vi "Digital Twin UI.vi"(8 "error in (no error)":errorcluster) -> (0 "error out":errorcluster)   [LabVIEW 2018]
uses:
  <vilib>/robotics/Controls/Simulator Display/Simulator Display.xctl
  Source Code_Headless/TestExec.llb/State Selector.ctl
  <vilib>/robotics/Simulator/Engine/ctl/Step Mode.ctl
  Source Code_Headless/TestExec.llb/TestStand UI Data.ctl
  <vilib>/NI Veristand/Execution/Workspace/NI VeriStand - Get Multiple Channel Values.vi
  <instrlib>/DC Motor Controller/HAIOL/DC Motor Controller.lvclass
  <vilib>/robotics/Simulator/NI_Robotics_Simulator.lvlib
  <instrlib>/DC Motor Controller/HAIOL/Simulator/DC Motor Controller Simulator.lvclass
  Source Code_Headless/TestExec.llb/TestStand Simple UI Dependencies.lvlib
  <vilib>/NI Veristand/Execution/Workspace/NI_VS Workspace ExecutionAPI.lvlib
  <vilib>/vision/driver/NI_Vision_Acquisition_Software.lvlib
  <resource>/objmgr/imaqdx.rc
panel:
  out "Enum":T1
  in  "TestStand UI Button Control":refnum<k7>(container)
  out "Numeric 2":i32
  out "DemoStop":bool
  out "DemoStart":bool
  out "Numeric":i32
  out "读数停止":bool
  out "Real Gear Position":T2(plugin-control)
  out "Time Stamp Control":timestamp format="%<%Y/%m/%d %X>T"
  out "WFC":dbl[][](graph)
  out "WFC - error":dbl[][](graph)
  out "Real Gear Enabled":bool
  out "Command":u16(ring) items=["抬起，Up，↑↑↑", "放下，Down，↓↓↓", "关闭，close，→→→"]
  out "WFC - torque":dbl(graph)
  out "Position Error:":dbl format="%#g deg"
  out "Sim Gear N Position:":dbl format="%#g deg"
  out "Real Gear N Position:":dbl format="%#g deg"
  out "LGCU Torque DutyCycle:":dbl format="%#g"
  out "Bypass Torque Calibration":bool
  out "Bypass Position Calibration":bool
  out "Sim Gear Position [deg]":dbl(slide) scale=0.0..180.0
  in  "Application Manager":refnum<k7>(container)
  in  "SequenceFileView Manager":refnum<k7>(container)
  in  "ExecutionView Manager":refnum<k7>(container)
  in  "Simulator Display":refnum<vi>(xcontrol)
  in  "manifest filename":string="Robotics Environment Simulator.xml"
  # "Digital Twin Demo -- Landing Gear Test"
  # "Gear Model"
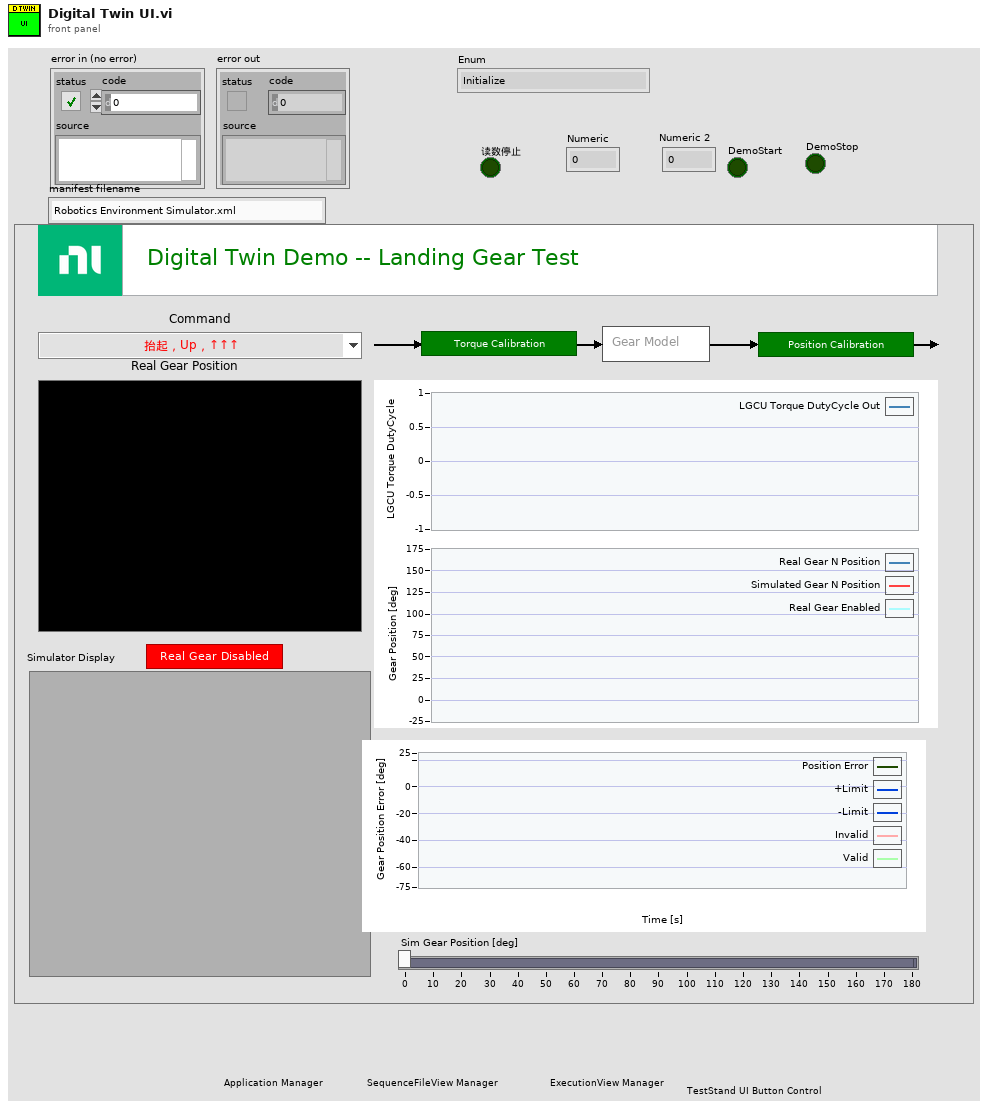
[diagram p1: front panel]
types:
  T1 = typedef "TestStand Simple UI Dependencies.lvlib/State Selector.ctl" = enum16{"Initialize", "Configure Connections", "Register Event Callbacks", "Start Application", "Execute", "Wait", "Stop", "Shutdown", "Handle Errors"}
  T2 = typedef "IMAQ Image.ctl" = refnum<image>
  T3 = typedef "TestStand Simple UI Dependencies.lvlib/TestStand UI Data.ctl" = cluster{"Other References":cluster{"Event Callback":refnum<k27>, "Quit Application Event":refnum<user-event>, "Event Reg Refnum":refnum<event-registration>, "Top level VI":refnum<vi>, "TestStand Engine":refnum<k7>}, "Manager Controls":cluster{"Application Manager":refnum<k7>, "SequenceFileView Manager":refnum<k7>, "ExecutionView Manager":refnum<k7>}, "Visible Controls":cluster{"Exit Button":refnum<k7>}}
  T4 = cluster{"Robot ID":string, "Device Label":string}
  T5 = typedef "NI_Robotics_Simulator.lvlib/Step Mode.ctl" = u16
  T6 = enum32{"invalid app kind", "Development System", "Run Time System", "Student Edition", "Embedded LabVIEW", "Evaluation", "Custom"}
  T7 = typedef "NI_VS Workspace ExecutionAPI.lvlib/WorkspaceAPI.ctl" = refnum<k24>
  T8 = typedef "IMAQdx.ctl" = refnum<k21>
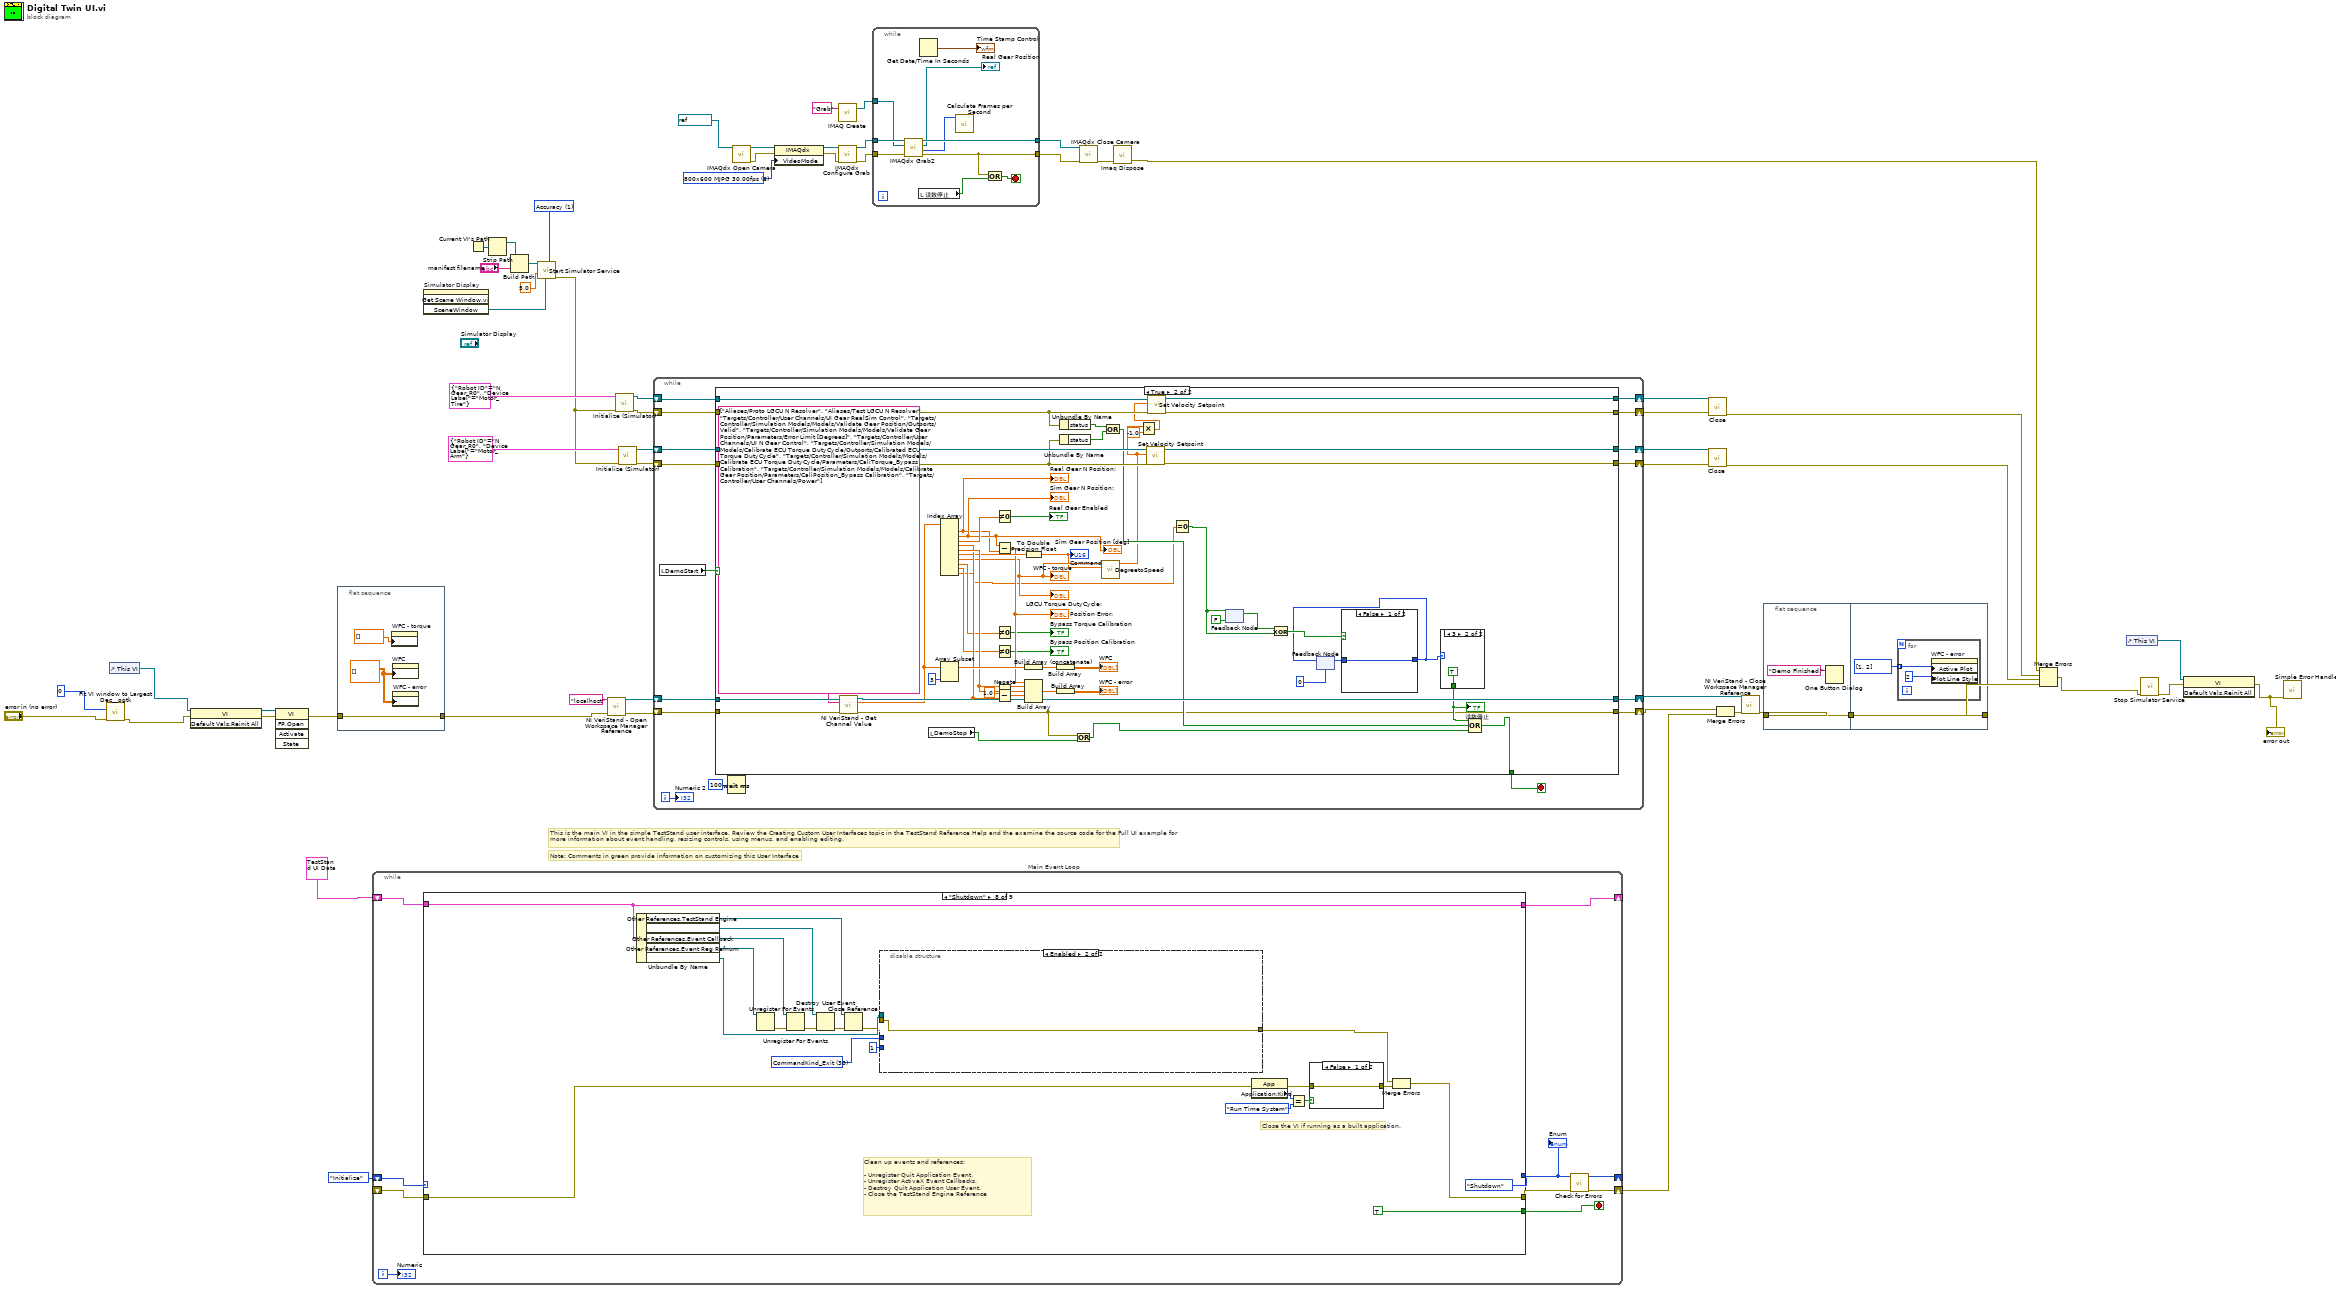
[diagram p0: block diagram]
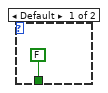
[diagram p3: hidden frame]
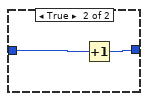
[diagram p4: hidden frame]
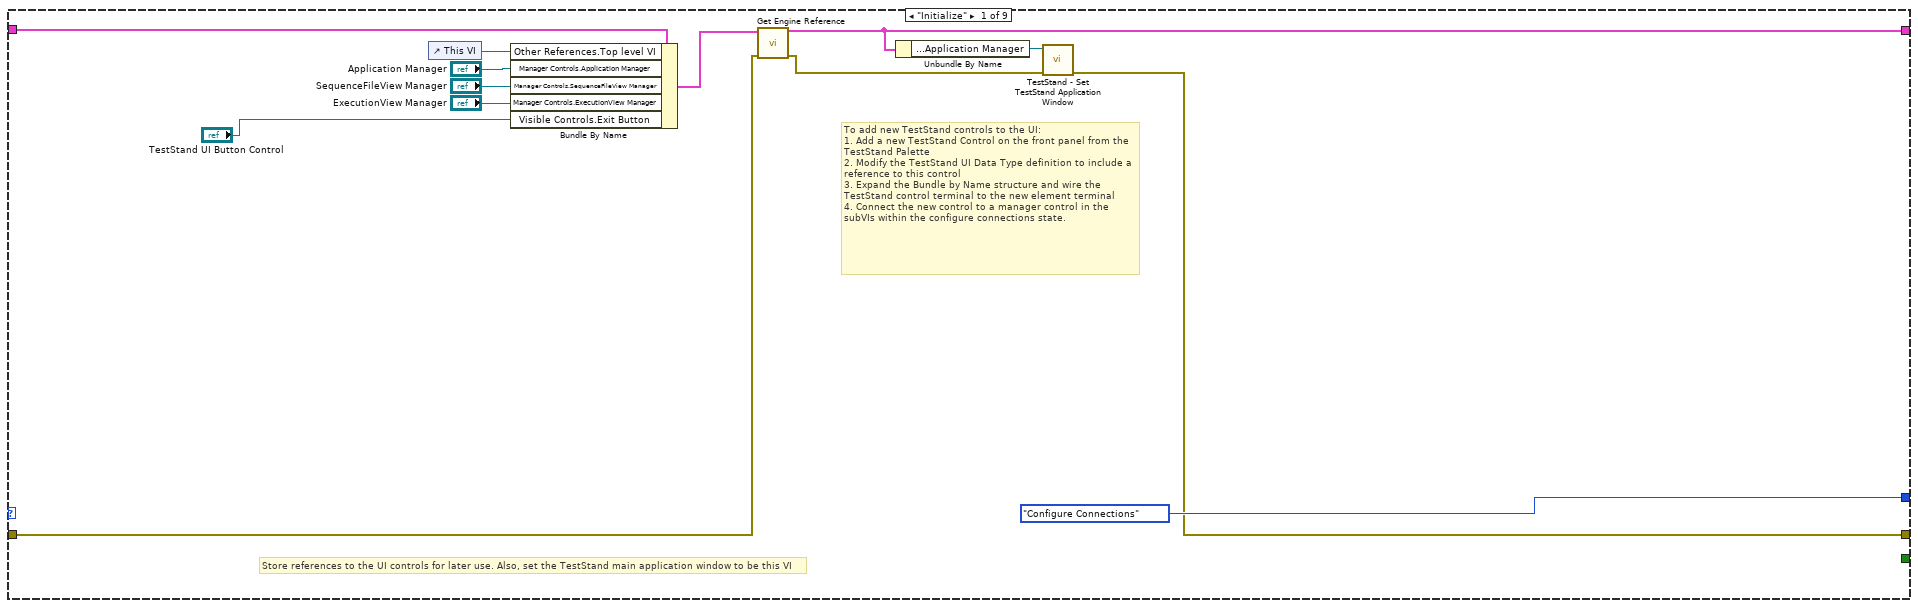
[diagram p5: hidden frame]
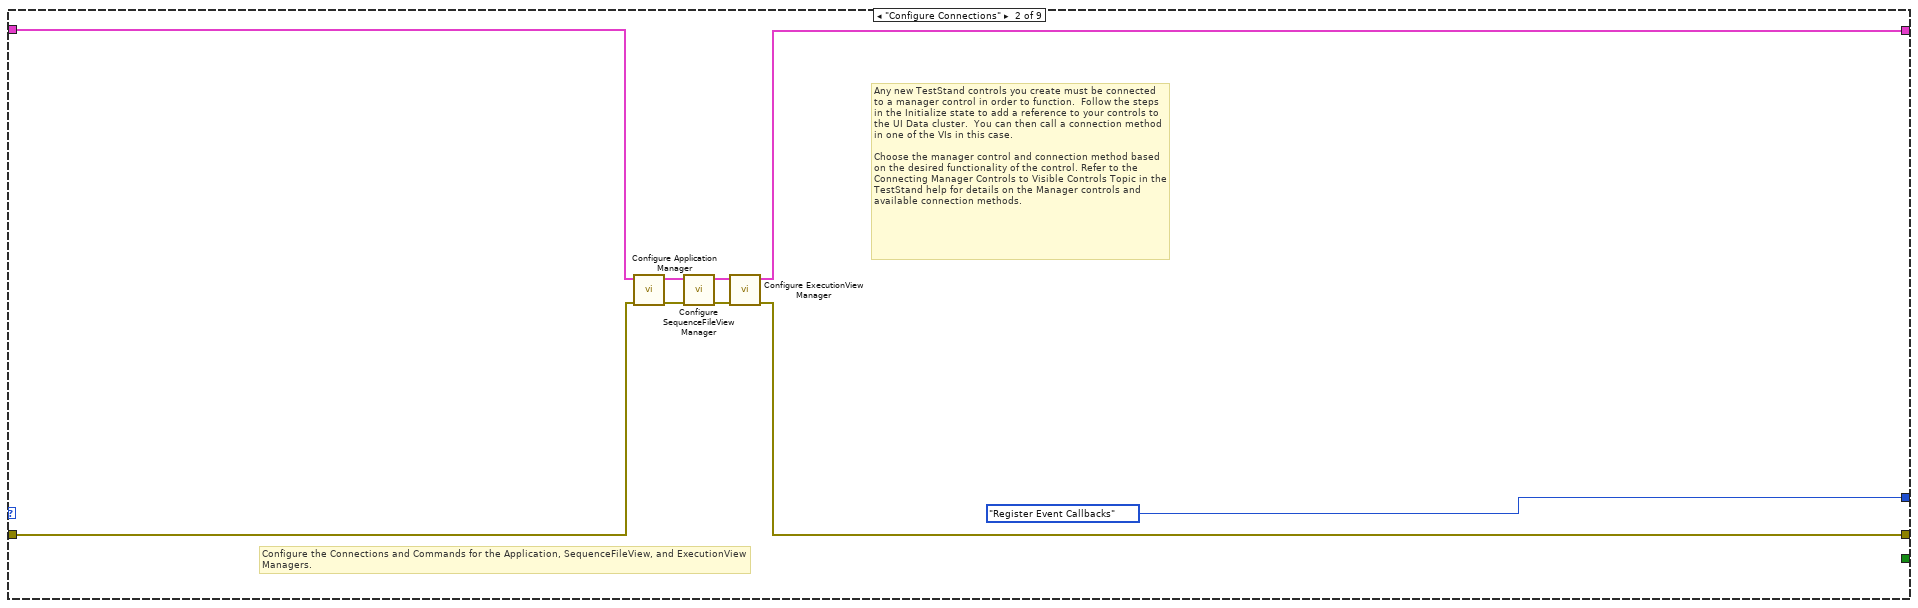
[diagram p6: hidden frame]
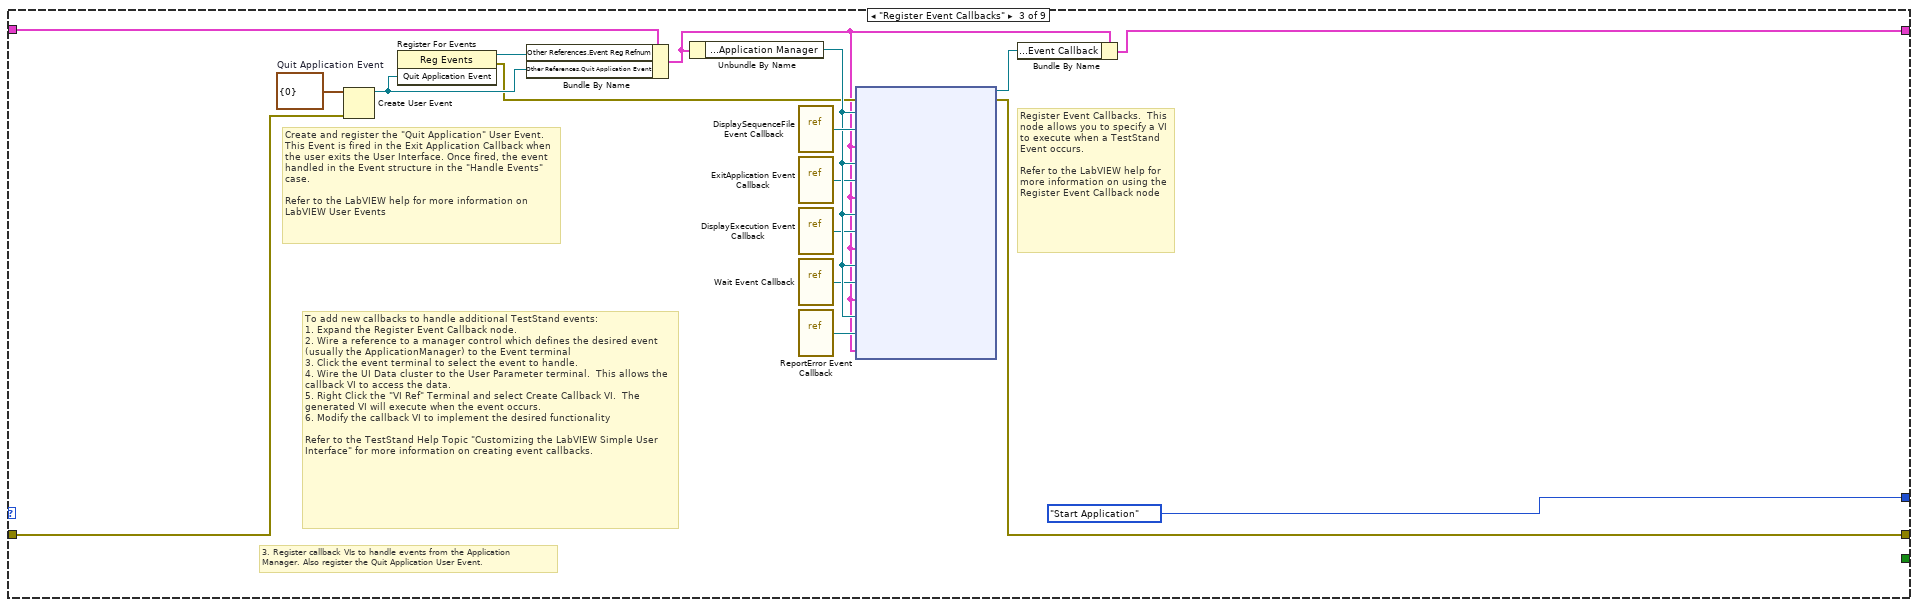
[diagram p7: hidden frame]
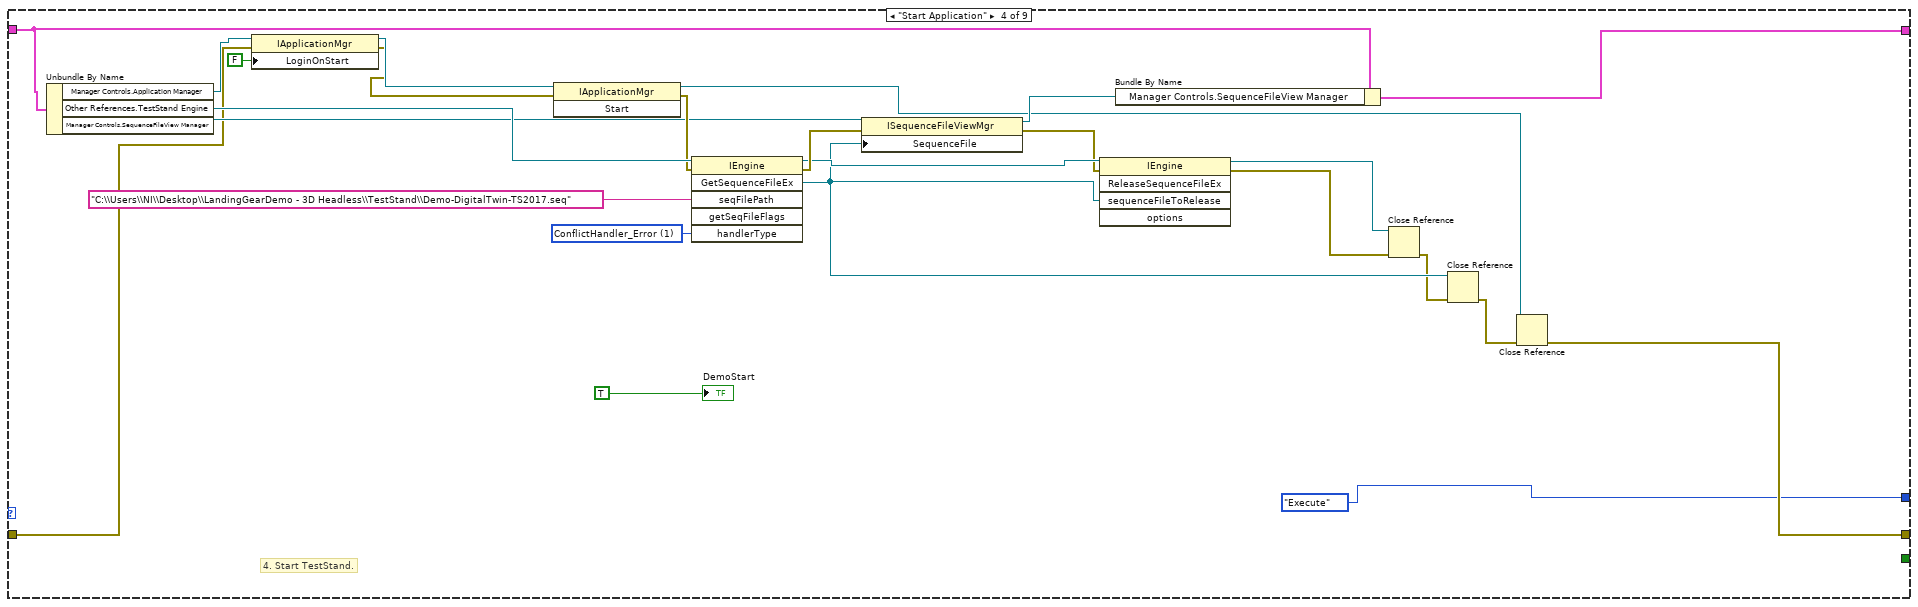
[diagram p8: hidden frame]
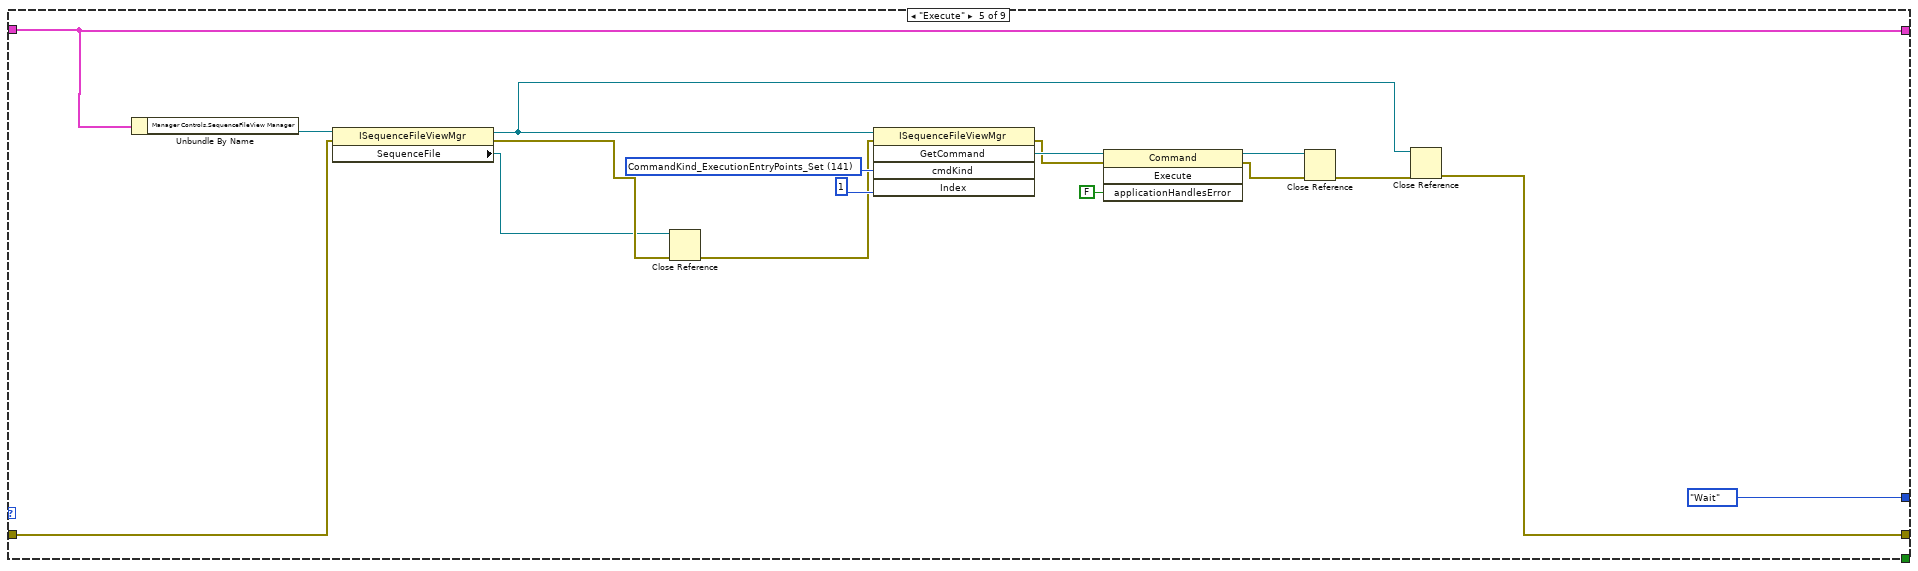
[diagram p9: hidden frame]
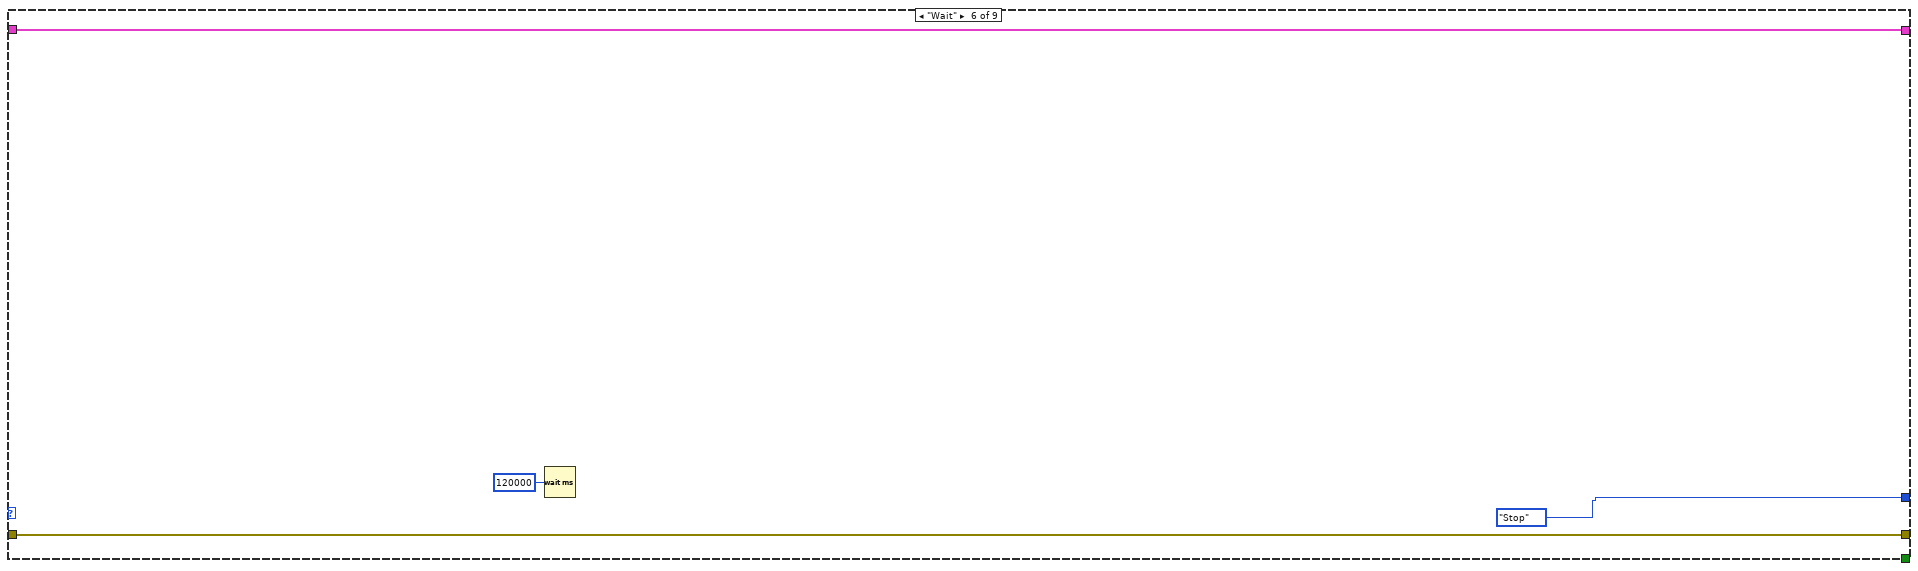
[diagram p10: hidden frame]
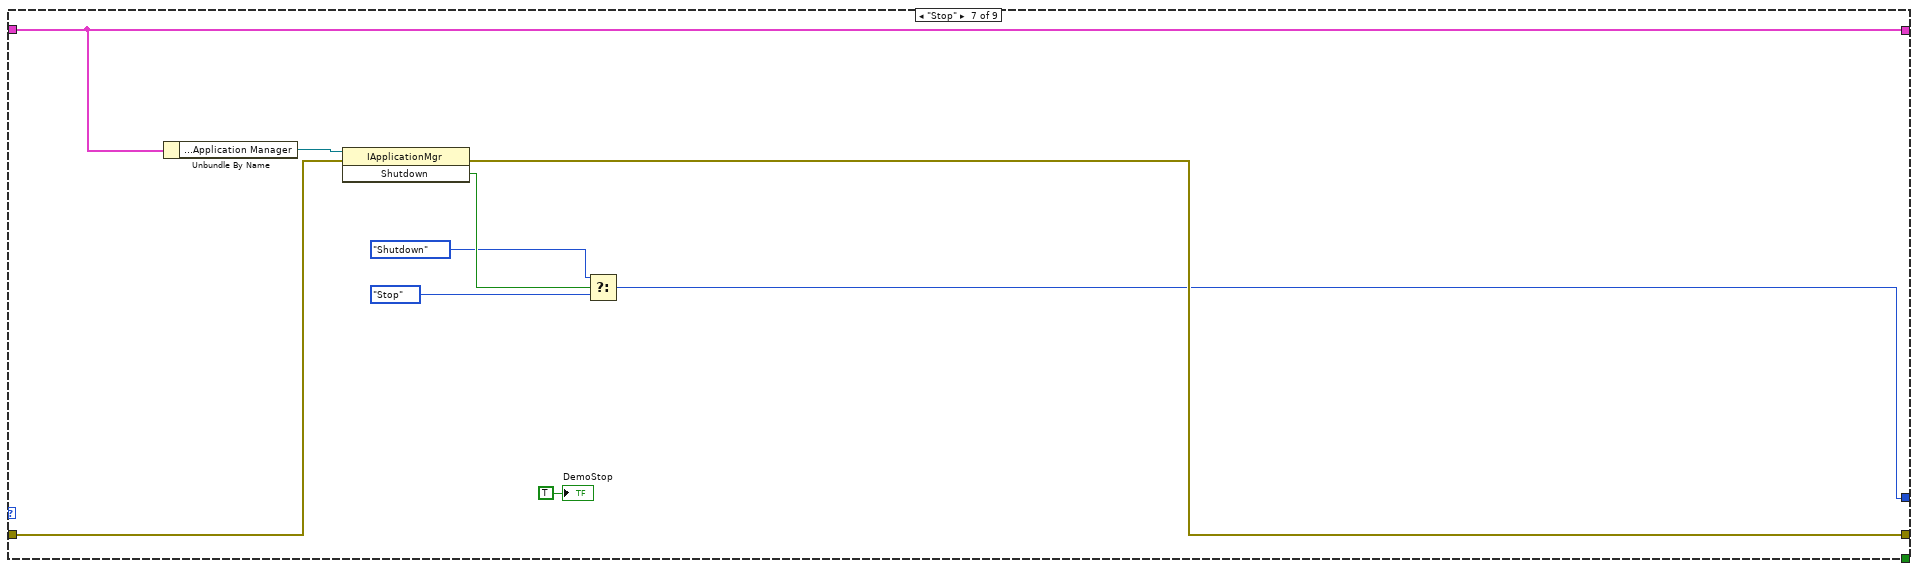
[diagram p11: hidden frame]
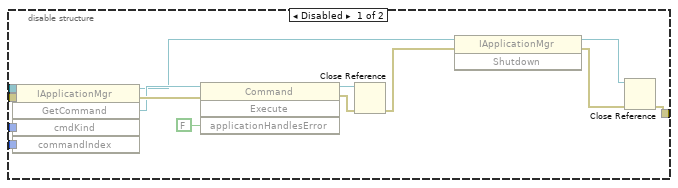
[diagram p12: hidden frame]
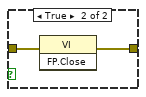
[diagram p13: hidden frame]
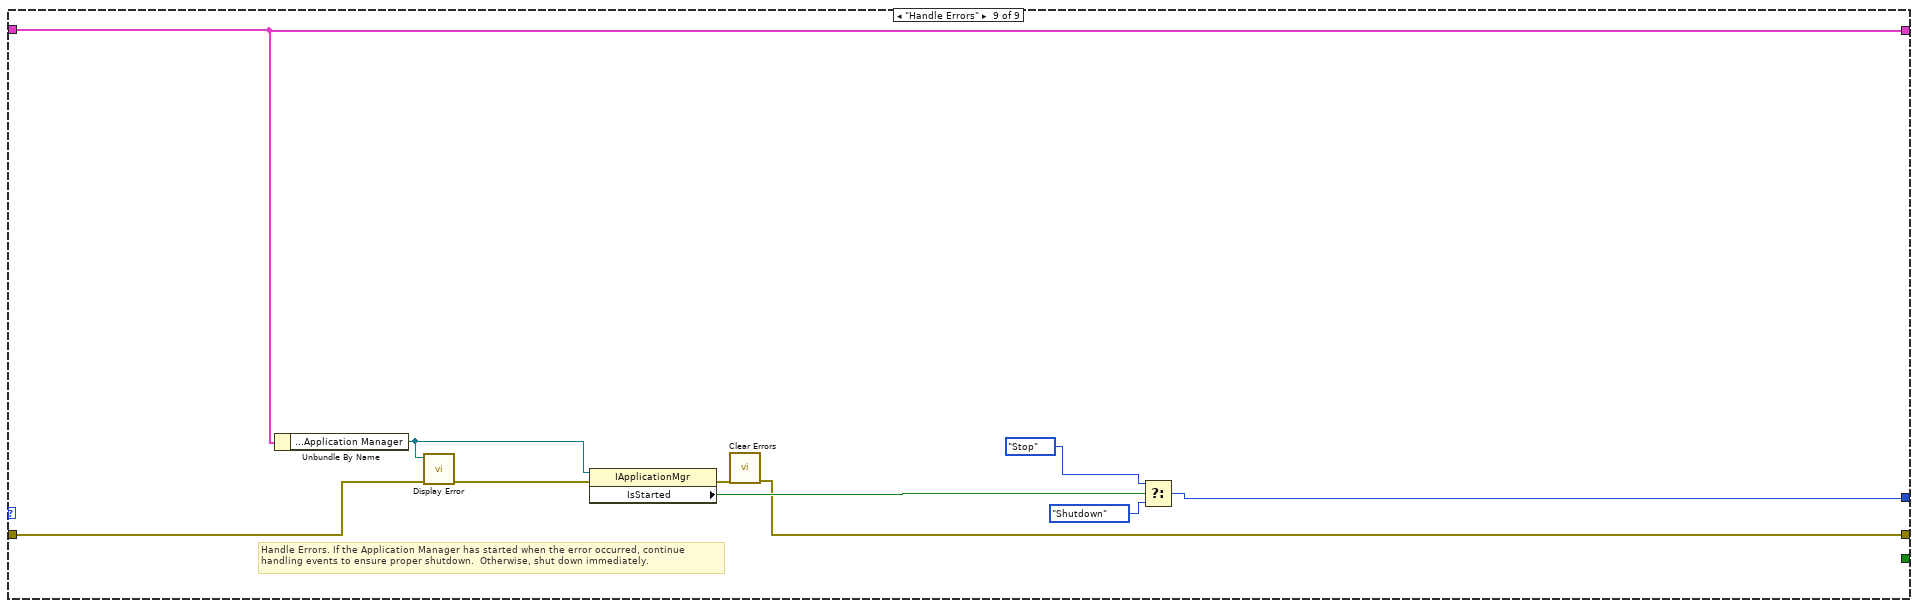
[diagram p14: hidden frame]
diagram:
  w28 = u32 6 items=["320x240 MJPG 30.00fps", "320x240 YUY2 30.00fps", "352x288 MJPG 30.00fps", "352x288 YUY2 30.00fps", "640x480 MJPG 30.00fps", "640x480 YUY2 30.00fps", "800x600 MJPG 30.00fps", "800x600 YUY2 30.00fps", "1024x768 MJPG 30.00fps", "1024x768 YUY2 10.00fps", "1280x720 MJPG 30.00fps", "1280x720 YUY2 10.00fps", "1920x1080 MJPG 30.00fps", "1920x1080 YUY2 5.00fps"] ("Video Modes")
  w50 = T5 1 items=["Performance", "Accuracy"] ("step mode")
  # "Note: Comments in green provide information on customizing this User Interface"
  # "This is the main VI in the simple TestStand user interface. Review the Creating Custom User Interfaces topic in the TestStand Reference Help and the examine the source code for the Full UI example for more information about event handling, resizing controls, using menus, and enabling editing."
  n1 = call <userlib>:"Fit VI window to Largest Dec__ogtk.vi"("error in (no error)"="error in (no error)", "border spacing (2 px)"=0) -> ("error out"=w13:errorcluster)  [unwired: 4 in, 1 out]
  n2 = control-ref of="This VI"() -> (w12:refnum<vi>)
  n3 = invoke class="VI" method="Default Vals.Reinit All"(reference=w12, error in=w13) -> (reference out=w11:refnum<vi>, error out=w14:errorcluster)  [unwired: 1 in, 1 out]
  n4 = invoke class="VI" method="FP.Open"(reference=w11, error in=w14) -> (error out=w58:errorcluster)  [unwired: 3 in, 4 out]
  n5 = flat-sequence {
    tunnel: [w61] -> w2
    tunnel: w58 -> [w61]
    frame #0 {
      w59 = dbl[][] [] ("History Data")
      n6 = property on="WFC - torque" class="WFChart (strict)"("History Data"=dbl[] []) -> ()  [unwired: 2 in, 2 out]
      n7 = property on="WFC" class="WFChart (strict)"("History Data"=w59) -> ()  [unwired: 2 in, 2 out]
      n8 = property on="WFC - error" class="WFChart (strict)"("History Data"=w59) -> ()  [unwired: 2 in, 2 out]
    }
  }
  n9 = while "Main Event Loop" {
    shift-right: [w64] -> w3
    shift-left: _ -> [w71]
    shift-right: [w65] -> _
    shift-left: State_Selector."Initialize" ("Enum") -> [w68]
    shift-right: [w70] -> _
    shift-left: T3 {"Other References"={"Event Callback"=refnum, "Quit Application Event"=refnum, "Event Reg Refnum"=refnum, "Top level VI"=refnum, "TestStand Engine"=refnum}, "Manager Controls"={"Application Manager"=refnum, "SequenceFileView Manager"=refnum, "ExecutionView Manager"=refnum}, "Visible Controls"={"Exit Button"=refnum}} ("TestStand UI Data") -> [w69]
    i -> [w62]
    stop <- w67 stop-if-true
    n10 = case shown="\"Shutdown\"" w68 {
      tunnel: w71 -> [w80 w89 w109 w120 w149 w153 w162 w171 w215]
      tunnel: [w76 w86 w95 w113 w145 w153 w161 w172 w207] -> w63
      tunnel: [w78 w85 w107 w126 w152 w156 w165 w182 w214] -> w70
      tunnel: w69 -> [w74 w90 w97 w127 w152 w156 w165 w182 w214]
      tunnel: [State_Selector."Configure Connections" ("Enum") State_Selector."Register Event Callbacks" ("Enum") State_Selector."Start Application" ("Enum") State_Selector."Execute" ("Enum") State_Selector."Wait" ("Enum") State_Selector."Stop" ("Enum") w158 State_Selector."Shutdown" ("Enum") w209] -> w66
      tunnel: [_ _ _ _ _ _ _ TRUE ("ShutDown") _] -> w67
      frame "Initialize" {
        # "To add new TestStand controls to the UI:\n1. Add a new TestStand Control on the front panel from the TestStand Palette \n2. Modify the TestStand UI Data Type definition to include a reference to this control\n3. Expand the Bundle by Name structure and wire the TestStand control terminal to the new element terminal\n4. Connect the new control to a manager control in the subVIs within the configure connections state."
        # "Store references to the UI controls for later use. Also, set the TestStand main application window to be this VI"
        n11 = control-ref of="This VI"() -> (w82:refnum<vi>)
        n12 = Bundle By Name(cluster=w74, "Other References.Top level VI"=w82, "Manager Controls.Application Manager"="Application Manager", "Manager Controls.SequenceFileView Manager"="SequenceFileView Manager", "Manager Controls.ExecutionView Manager"="ExecutionView Manager", "Visible Controls.Exit Button"="TestStand UI Button Control") -> (w73:T3)
        n13 = call "Get Engine Reference.vi"("error in (no error)"=w80, "TestStand UI Data In"=w73) -> ("error out"=w77:errorcluster, "TestStand UI Data Out"=w78:T3)  [unwired: 8 in]
        n14 = Unbundle By Name(w78) -> ("Manager Controls.Application Manager"=w79:refnum<k7>)
        n15 = call <vilib>:"TestStand - Set TestStand Application Window.vi"("error in (no error)"=w77, "Application Manager"=w79) -> ("error out"=w76:errorcluster)  [unwired: 1 in, 8 out]
      }
      frame "Configure Connections" {
        # "Any new TestStand controls you create must be connected to a manager control in order to function.  Follow the steps in the Initialize state to add a reference to your controls to the UI Data cluster.  You can then call a connection method in one of the VIs in this case.  \n\nChoose the manager control and connection method based on the desired functionality of the control. Refer to the Connecting Manager Controls to Visible Controls Topic in the TestStand help for details on the Manager controls and available connection methods."
        # "Configure the Connections and Commands for the Application, SequenceFileView, and ExecutionView Managers."
        n16 = call "Configure Application Manager.vi"("error in (no error)"=w89, "TestStand Controls"=w90) -> ("error out"=w93:errorcluster, "TestStand Controls Out"=w91:T3)  [unwired: 1 in, 7 out]
        n17 = call "Configure SequenceFileView Manager.vi"("error in (no error)"=w93, "TestStand Controls"=w91) -> ("error out"=w87:errorcluster, "TestStand Controls Out"=w88:T3)  [unwired: 8 in]
        n18 = call "Configure ExecutionView Manager.vi"("error in (no error)"=w87, "TestStand Controls"=w88) -> ("error out"=w86:errorcluster, "TestStand Controls Out"=w85:T3)  [unwired: 6 in, 2 out]
      }
      frame "Register Event Callbacks" {
        w110 = cluster{"Number":i32} {"Number"=0}  # Quit Application Event
        # "Register Event Callbacks.  This node allows you to specify a VI to execute when a TestStand Event occurs. \n\nRefer to the LabVIEW help for more information on using the Register Event Callback node"
        # "Create and register the \"Quit Application\" User Event. This Event is fired in the Exit Application Callback when the user exits the User Interface. Once fired, the event handled in the Event structure in the \"Handle Events\" case.\n\nRefer to the LabVIEW help for more information on LabVIEW User Events"
        # "To add new callbacks to handle additional TestStand events:\n1. Expand the Register Event Callback node.  \n2. Wire a reference to a manager control which defines the desired event (usually the ApplicationManager) to the Event terminal\n3. Click the event terminal to select the event to handle.\n4. Wire the UI Data cluster to the User Parameter terminal.  This allows the callback VI to access the data.\n5. Right Click the \"VI Ref\" Terminal and select Create Callback VI.  The generated VI will execute when the event occurs.\n6. Modify the callback VI to implement the desired functionality\n\nRefer to the TestStand Help Topic \"Customizing the LabVIEW Simple User Interface\" for more information on creating event callbacks."
        # "3. Register callback VIs to handle events from the Application\nManager. Also register the Quit Application User Event."
        n19 = Create User Event(user event datatype=w110, error in=w109) -> (user event=w99:refnum<user-event>)  [unwired: 1 out]
        n20 = register-events(w99) -> (reference out=w98:refnum<event-registration>, error out=w96:errorcluster)  [unwired: 2 in]
        n21 = Bundle By Name(cluster=w97, "Other References.Event Reg Refnum"=w98, "Other References.Quit Application Event"=w99) -> (w94:T3)
        n22 = Unbundle By Name(w94) -> ("Manager Controls.Application Manager"=w104:refnum<k7>)
        n23 = vi-ref "DisplaySequenceFile Event Callback.vi"() -> ("vi reference"=w105:refnum<vi>)
        n24 = vi-ref "ExitApplication Event Callback.vi"() -> ("vi reference"=w102:refnum<vi>)
        n25 = vi-ref "DisplayExecution Event Callback.vi"() -> ("vi reference"=w101:refnum<vi>)
        n26 = vi-ref "Wait Event Callback.vi"() -> ("vi reference"=w100:refnum<vi>)
        n27 = vi-ref "ReportError Event Callback.vi"() -> ("vi reference"=w103:refnum<vi>)
        n28 = node(w96, w104, w105, w94, w104, w102, w94, w104, w101, w94, w104, w100, w94, w104, w103, w94) -> (w106:refnum<k27>, w95:errorcluster)  [unwired: 1 in]
        n29 = Bundle By Name(cluster=w94, "Other References.Event Callback"=w106) -> (w107:T3)
      }
      frame "Start Application" {
        w133 = 1 items=["ConflictHandler_Error"=1, "ConflictHandler_Prompt"=3, "ConflictHandler_UseGlobalType"=4] ("handlerType")
        # "4. Start TestStand."
        n30 = Unbundle By Name(w127) -> ("Manager Controls.Application Manager"=w123:refnum<k7>, "Other References.TestStand Engine"=w135:refnum<k7>, "Manager Controls.SequenceFileView Manager"=w132:refnum<k7>)
        n31 = property class="IApplicationMgr"(reference=w123, error in=w120, "LoginOnStart"=FALSE) -> (reference out=w121:refnum<k7>, error out=w119:errorcluster)
        n32 = invoke class="IApplicationMgr" method="Start"(reference=w121, error in=w119) -> (reference out=w115:refnum<k7>, error out=w134:errorcluster)  [unwired: 1 in, 1 out]
        n33 = invoke class="IEngine" method="GetSequenceFileEx"(reference=w135, error in=w134, "seqFilePath"="C:\\Users\\NI\\Desktop\\LandingGearDemo - 3D Headless\\TestStand\\Demo-DigitalTwin-TS2017.seq", "handlerType"=w133) -> (reference out=w130:refnum<k7>, error out=w131:errorcluster, "GetSequenceFileEx"=w125:refnum<k7>)  [unwired: 2 in, 3 out]
        n34 = property class="ISequenceFileViewMgr"(reference=w132, error in=w131, "SequenceFile"=w125) -> (reference out=w128:refnum<k7>, error out=w129:errorcluster)
        n35 = invoke class="IEngine" method="ReleaseSequenceFileEx"(reference=w130, error in=w129, "sequenceFileToRelease"=w125) -> (reference out=w118:refnum<k7>, error out=w117:errorcluster)  [unwired: 2 in, 3 out]
        n36 = Bundle By Name(cluster=w127, "Manager Controls.SequenceFileView Manager"=w128) -> (w126:T3)
        n37 = Close Reference(reference=w118, error in (no error)=w117) -> (error out=w116:errorcluster)
        n38 = Close Reference(reference=w125, error in (no error)=w116) -> (error out=w114:errorcluster)
        n39 = Close Reference(reference=w115, error in (no error)=w114) -> (error out=w113:errorcluster)
        "DemoStart" <- TRUE
      }
      frame "Execute" {
        w143 = 141 items=["CommandKind_NotACommand"=0, "CommandKind_Container"=1, "CommandKind_Separator"=2, "CommandKind_Custom"=3, "CommandKind_OpenSequenceFile"=20, "CommandKind_Close"=21, "CommandKind_CloseAll"=22, "CommandKind_CloseCompletedExecutions"=23, "CommandKind_OpenWorkspaceBrowser"=24, "CommandKind_Login"=25, "CommandKind_Logout"=26, "CommandKind_LoginLogout"=27, "CommandKind_UnloadAllModules"=28, "CommandKind_MRUFile"=29, "CommandKind_Exit"=30, "CommandKind_Restart"=40, "CommandKind_RunEntryPoint"=41, "CommandKind_RunEntryPointOnSelectedSteps"=42, "CommandKind_LoopEntryPointOnSelectedSteps"=43, "CommandKind_RunCurrentSequence"=44, "CommandKind_RunSpecificSequence"=45, "CommandKind_RunSelectedSteps"=46, "CommandKind_RunSelectedStepsUsingEntryPointsSubmenu"=47, "CommandKind_LoopOnSelectedSteps"=48, "CommandKind_LoopOnSelectedStepsUsingEntryPointsSubmenu"=49, "CommandKind_BreakOnFirstStep"=50, "CommandKind_BreakOnStepFailure"=51, "CommandKind_BreakOnSequenceFailure"=52, "CommandKind_TracingEnabled"=53, "CommandKind_ToggleBreakpoint"=60, "CommandKind_SetRunModeSubmenu"=61, "CommandKind_RunModeForcePass"=62, "CommandKind_RunModeForceFail"=63, "CommandKind_RunModeSkip"=64, "CommandKind_RunModeNormal"=65, "CommandKind_Resume"=66, "CommandKind_StepInto"=67, "CommandKind_StepOver"=68, "CommandKind_StepOut"=69, "CommandKind_SetNextStep"=70, "CommandKind_Break"=71, "CommandKind_BreakResume"=72, "CommandKind_Terminate"=73, "CommandKind_TerminateRestart"=74, "CommandKind_Abort"=75, "CommandKind_BreakAll"=76, "CommandKind_TerminateAll"=77, "CommandKind_AbortAll"=78, "CommandKind_ResumeAll"=79, "CommandKind_DisplayBreakpointsAndWatchExpressions"=80, "CommandKind_DisplayBreakpointSettings"=81, "CommandKind_BreakpointSubmenu"=85, "CommandKind_ConfigureAdapters"=90, "CommandKind_ConfigureStationOptions"=91, "CommandKind_ConfigureSearchDirectories"=92, "CommandKind_ConfigureExternalViewers"=93, "CommandKind_ConfigureEngineEnvironment"=94, "CommandKind_ToolItem"=100, "CommandKind_CustomizeTools"=101, "CommandKind_ExecutionEntryPointInsertionMarker"=110, "CommandKind_ExecutionEntryPointDefaultMenuInsertionMarker"=111, "CommandKind_ConfigurationEntryPointInsertionMarker"=112, "CommandKind_ConfigurationEntryPointDefaultMenuInsertionMarker"=113, "CommandKind_SequenceViewConfiguration"=116, "CommandKind_SequenceViewConfigurationsSubmenu"=118, "CommandKind_DefaultFileMenu_Set"=120, "CommandKind_DefaultExecuteMenu_Set"=121, "CommandKind_DefaultDebugMenu_Set"=123, "CommandKind_DefaultConfigureMenu_Set"=124, "CommandKind_DefaultToolsMenu_Set"=125, "CommandKind_DefaultSequenceViewContextMenu_Set"=126, "CommandKind_DefaultListBarContextMenu_Set"=127, "CommandKind_DefaultEditMenu_Set"=128, "CommandKind_DefaultSequenceListContextMenu_Set"=129, "CommandKind_SequenceViewConfigurations_Set"=139, "CommandKind_MRUFiles_Set"=140, "CommandKind_ExecutionEntryPoints_Set"=141, "CommandKind_RunSequences_Set"=142, "CommandKind_RunSelectedStepsUsingEntryPoints_Set"=143, "CommandKind_LoopOnSelectedStepsUsingEntryPoints_Set"=144, "CommandKind_ConfigurationEntryPoints_Set"=145, "CommandKind_Tools_Set"=146, "CommandKind_OpenSequenceFiles"=147, "CommandKind_LockUnlock"=148, "CommandKind_ConfigureSequenceViews"=149, "CommandKind_Edit_Undo"=200, "CommandKind_Edit_Redo"=201, "CommandKind_Edit_Rename"=202, "CommandKind_Edit_Cut"=203, "CommandKind_Edit_Copy"=204, "CommandKind_Edit_Paste"=205, "CommandKind_Edit_Delete"=206, "CommandKind_Edit_InsertStep"=207, "CommandKind_Edit_Save"=208, "CommandKind_Edit_SaveAs"=209, "CommandKind_Edit_SaveAll"=210, "CommandKind_Edit_NewSequenceFile"=211, "CommandKind_Edit_StepProperties"=212, "CommandKind_Edit_SequenceProperties"=213, "CommandKind_Edit_SequenceFileProperties"=214, "CommandKind_Edit_SpecifyModule"=215, "CommandKind_Edit_EditCode"=216, "CommandKind_Edit_EditStep"=217, "CommandKind_Edit_Preconditions"=218, "CommandKind_SelectAll"=219, "CommandKind_Edit_SelectDefaultAdapter"=220, "CommandKind_Edit_InsertSequence"=221, "CommandKind_Edit_SequenceFileCallbacks"=222, "CommandKind_Edit_EditPaths"=223, "CommandKind_Edit_EncapsulateSelectedSteps"=224, "CommandKind_Edit_InsertStepsSubmenu"=300, "CommandKind_Edit_EditStepsSubmenu"=301, "CommandKind_Edit_SelectDefaultAdaptersSubmenu"=302, "CommandKind_Edit_EncapsulateSelectedStepsSubmenu"=303, "CommandKind_Edit_InsertSteps_Set"=340, "CommandKind_Edit_EditSteps_Set"=341, "CommandKind_Edit_SelectDefaultAdapters_Set"=342, "CommandKind_Edit_EncapsulateSelectedSteps_Set"=343, "CommandKind_ShowInList"=400, "CommandKind_ShowInVariables"=401, "CommandKind_ShowTestStandHelp"=420, "CommandKind_ShowGuideToDocumentation"=421, "CommandKind_ShowHelpTopic"=422, "CommandKind_ShowTestStandWebResources"=423, "CommandKind_ShowTestStandDiscussionForum"=424, "CommandKind_ShowPatents"=425, "CommandKind_DefaultHelpMenu_Set"=440, "CommandKind_Edit_Attributes"=450, "CommandKind_Edit_AdvancedSequenceListSubmenu"=451, "CommandKind_ShowUpdateService"=452, "CommandKind_ShowExamples"=453, "CommandKind_ShowGettingStarted"=454, "CommandKind_UnloadStepModule"=455] ("cmdKind")
        n40 = Unbundle By Name(w152) -> ("Manager Controls.SequenceFileView Manager"=w151:refnum<k7>)
        n41 = property class="ISequenceFileViewMgr"(reference=w151, error in=w149) -> (reference out=w146:refnum<k7>, error out=w148:errorcluster, "SequenceFile"=w147:refnum<k7>)
        n42 = Close Reference(reference=w147, error in (no error)=w148) -> (error out=w136:errorcluster)
        n43 = invoke class="ISequenceFileViewMgr" method="GetCommand"(reference=w146, error in=w136, "cmdKind"=w143, "Index"=1) -> (error out=w138:errorcluster, "GetCommand"=w141:refnum<k7>)  [unwired: 1 in, 3 out]
        n44 = invoke class="Command" method="Execute"(reference=w141, error in=w138, "applicationHandlesError"=FALSE) -> (reference out=w139:refnum<k7>, error out=w137:errorcluster)  [unwired: 1 in, 2 out]
        n45 = Close Reference(reference=w139, error in (no error)=w137) -> (error out=w150:errorcluster)
        n46 = Close Reference(reference=w146, error in (no error)=w150) -> (error out=w145:errorcluster)
      }
      frame "Wait" {
        n47 = Wait (ms)(milliseconds to wait=u32 120000) -> ()  [unwired: 1 out]
      }
      frame "Stop" {
        n48 = Unbundle By Name(w165) -> ("Manager Controls.Application Manager"=w164:refnum<k7>)
        n49 = invoke class="IApplicationMgr" method="Shutdown"(reference=w164, error in=w162) -> (error out=w161:errorcluster, "Shutdown"=w163:bool)  [unwired: 1 in, 1 out]
        n50 = Select(t=State_Selector."Shutdown" ("Enum"), s=w163, f=State_Selector."Stop" ("Enum")) -> (s? t:f=w158:T1)
        "DemoStop" <- TRUE
      }
      frame "Shutdown" {
        w170 = 30 items=["CommandKind_NotACommand"=0, "CommandKind_Container"=1, "CommandKind_Separator"=2, "CommandKind_Custom"=3, "CommandKind_OpenSequenceFile"=20, "CommandKind_Close"=21, "CommandKind_CloseAll"=22, "CommandKind_CloseCompletedExecutions"=23, "CommandKind_OpenWorkspaceBrowser"=24, "CommandKind_Login"=25, "CommandKind_Logout"=26, "CommandKind_LoginLogout"=27, "CommandKind_UnloadAllModules"=28, "CommandKind_MRUFile"=29, "CommandKind_Exit"=30, "CommandKind_Restart"=40, "CommandKind_RunEntryPoint"=41, "CommandKind_RunEntryPointOnSelectedSteps"=42, "CommandKind_LoopEntryPointOnSelectedSteps"=43, "CommandKind_RunCurrentSequence"=44, "CommandKind_RunSpecificSequence"=45, "CommandKind_RunSelectedSteps"=46, "CommandKind_RunSelectedStepsUsingEntryPointsSubmenu"=47, "CommandKind_LoopOnSelectedSteps"=48, "CommandKind_LoopOnSelectedStepsUsingEntryPointsSubmenu"=49, "CommandKind_BreakOnFirstStep"=50, "CommandKind_BreakOnStepFailure"=51, "CommandKind_BreakOnSequenceFailure"=52, "CommandKind_TracingEnabled"=53, "CommandKind_ToggleBreakpoint"=60, "CommandKind_SetRunModeSubmenu"=61, "CommandKind_RunModeForcePass"=62, "CommandKind_RunModeForceFail"=63, "CommandKind_RunModeSkip"=64, "CommandKind_RunModeNormal"=65, "CommandKind_Resume"=66, "CommandKind_StepInto"=67, "CommandKind_StepOver"=68, "CommandKind_StepOut"=69, "CommandKind_SetNextStep"=70, "CommandKind_Break"=71, "CommandKind_BreakResume"=72, "CommandKind_Terminate"=73, "CommandKind_TerminateRestart"=74, "CommandKind_Abort"=75, "CommandKind_BreakAll"=76, "CommandKind_TerminateAll"=77, "CommandKind_AbortAll"=78, "CommandKind_ResumeAll"=79, "CommandKind_DisplayBreakpointsAndWatchExpressions"=80, "CommandKind_DisplayBreakpointSettings"=81, "CommandKind_BreakpointSubmenu"=85, "CommandKind_ConfigureAdapters"=90, "CommandKind_ConfigureStationOptions"=91, "CommandKind_ConfigureSearchDirectories"=92, "CommandKind_ConfigureExternalViewers"=93, "CommandKind_ConfigureEngineEnvironment"=94, "CommandKind_ToolItem"=100, "CommandKind_CustomizeTools"=101, "CommandKind_ExecutionEntryPointInsertionMarker"=110, "CommandKind_ExecutionEntryPointDefaultMenuInsertionMarker"=111, "CommandKind_ConfigurationEntryPointInsertionMarker"=112, "CommandKind_ConfigurationEntryPointDefaultMenuInsertionMarker"=113, "CommandKind_SequenceViewConfiguration"=116, "CommandKind_SequenceViewConfigurationsSubmenu"=118, "CommandKind_DefaultFileMenu_Set"=120, "CommandKind_DefaultExecuteMenu_Set"=121, "CommandKind_DefaultDebugMenu_Set"=123, "CommandKind_DefaultConfigureMenu_Set"=124, "CommandKind_DefaultToolsMenu_Set"=125, "CommandKind_DefaultSequenceViewContextMenu_Set"=126, "CommandKind_DefaultListBarContextMenu_Set"=127, "CommandKind_DefaultEditMenu_Set"=128, "CommandKind_DefaultSequenceListContextMenu_Set"=129, "CommandKind_SequenceViewConfigurations_Set"=139, "CommandKind_MRUFiles_Set"=140, "CommandKind_ExecutionEntryPoints_Set"=141, "CommandKind_RunSequences_Set"=142, "CommandKind_RunSelectedStepsUsingEntryPoints_Set"=143, "CommandKind_LoopOnSelectedStepsUsingEntryPoints_Set"=144, "CommandKind_ConfigurationEntryPoints_Set"=145, "CommandKind_Tools_Set"=146, "CommandKind_OpenSequenceFiles"=147, "CommandKind_LockUnlock"=148, "CommandKind_ConfigureSequenceViews"=149, "CommandKind_Edit_Undo"=200, "CommandKind_Edit_Redo"=201, "CommandKind_Edit_Rename"=202, "CommandKind_Edit_Cut"=203, "CommandKind_Edit_Copy"=204, "CommandKind_Edit_Paste"=205, "CommandKind_Edit_Delete"=206, "CommandKind_Edit_InsertStep"=207, "CommandKind_Edit_Save"=208, "CommandKind_Edit_SaveAs"=209, "CommandKind_Edit_SaveAll"=210, "CommandKind_Edit_NewSequenceFile"=211, "CommandKind_Edit_StepProperties"=212, "CommandKind_Edit_SequenceProperties"=213, "CommandKind_Edit_SequenceFileProperties"=214, "CommandKind_Edit_SpecifyModule"=215, "CommandKind_Edit_EditCode"=216, "CommandKind_Edit_EditStep"=217, "CommandKind_Edit_Preconditions"=218, "CommandKind_SelectAll"=219, "CommandKind_Edit_SelectDefaultAdapter"=220, "CommandKind_Edit_InsertSequence"=221, "CommandKind_Edit_SequenceFileCallbacks"=222, "CommandKind_Edit_EditPaths"=223, "CommandKind_Edit_EncapsulateSelectedSteps"=224, "CommandKind_Edit_InsertStepsSubmenu"=300, "CommandKind_Edit_EditStepsSubmenu"=301, "CommandKind_Edit_SelectDefaultAdaptersSubmenu"=302, "CommandKind_Edit_EncapsulateSelectedStepsSubmenu"=303, "CommandKind_Edit_InsertSteps_Set"=340, "CommandKind_Edit_EditSteps_Set"=341, "CommandKind_Edit_SelectDefaultAdapters_Set"=342, "CommandKind_Edit_EncapsulateSelectedSteps_Set"=343, "CommandKind_ShowInList"=400, "CommandKind_ShowInVariables"=401, "CommandKind_ShowTestStandHelp"=420, "CommandKind_ShowGuideToDocumentation"=421, "CommandKind_ShowHelpTopic"=422, "CommandKind_ShowTestStandWebResources"=423, "CommandKind_ShowTestStandDiscussionForum"=424, "CommandKind_ShowPatents"=425, "CommandKind_DefaultHelpMenu_Set"=440, "CommandKind_Edit_Attributes"=450, "CommandKind_Edit_AdvancedSequenceListSubmenu"=451, "CommandKind_ShowUpdateService"=452, "CommandKind_ShowExamples"=453, "CommandKind_ShowGettingStarted"=454, "CommandKind_UnloadStepModule"=455] ("cmdKind")
        # "Close the VI if running as a built application."
        # "Clean up events and references:\n\n- Unregister Quit Application Event.\n- Unregister ActiveX Event Callbacks.\n- Destroy Quit Application User Event.\n- Close the TestStand Engine Reference"
        n51 = Unbundle By Name(w182) -> ("Other References.TestStand Engine"=w178:refnum<k7>, "Other References.Quit Application Event"=w180:refnum<user-event>, "Other References.Event Callback"=w183:refnum<k27>, "Other References.Event Reg Refnum"=w181:refnum<event-registration>, "Manager Controls.Application Manager"=w168:refnum<k7>)
        n52 = Unregister For Events(event registration refnum=w181) -> (error out=w184:errorcluster)  [unwired: 1 in]
        n53 = Unregister For Events(event registration refnum=w183, error in=w184) -> (error out=w185:errorcluster)
        n54 = Destroy User Event(user event=w180, error in=w185) -> (error out=w179:errorcluster)
        n55 = Close Reference(reference=w178, error in (no error)=w179) -> (error out=w167:errorcluster)
        n56 = disable-structure shown="Enabled" {
          disable-tunnel: w170 -> [w201 _]
          disable-tunnel: 1 ("commandIndex") -> [w200 _]
          disable-tunnel: w168 -> [w194 _]
          disable-tunnel: w167 -> [w193 w202]
          disable-tunnel: [w189 w202] -> w166
          frame Disabled {
            n57 = invoke class="IApplicationMgr" method="GetCommand"(reference=w194, error in=w193, "cmdKind"=w201, "commandIndex"=w200) -> (reference out=w192:refnum<k7>, error out=w199:errorcluster, "GetCommand"=w198:refnum<k7>)  [unwired: 1 in, 2 out]
            n58 = invoke class="Command" method="Execute"(reference=w198, error in=w199, "applicationHandlesError"=FALSE) -> (reference out=w196:refnum<k7>, error out=w195:errorcluster)  [unwired: 1 in, 2 out]
            n59 = Close Reference(reference=w196, error in (no error)=w195) -> (error out=w191:errorcluster)
            n60 = invoke class="IApplicationMgr" method="Shutdown"(reference=w192, error in=w191) -> (reference out=w188:refnum<k7>, error out=w190:errorcluster)  [unwired: 1 in, 1 out]
            n61 = Close Reference(reference=w188, error in (no error)=w190) -> (error out=w189:errorcluster)
          }
          frame Enabled {
          }
        }
        n62 = property class="App"(error in=w171) -> (error out=w174:errorcluster, "Application:Kind"=w176:T6)  [unwired: 1 in, 1 out]
        n63 = Equal?(x=w176, y=T6."Run Time System" ("Application:Kind")) -> (x = y?=w175:bool)
        n64 = case shown="False" w175 {
          tunnel: w174 -> [w203 w205]
          tunnel: [w203 w204] -> w173
          frame False {
          }
          frame True {
            n65 = invoke class="VI" method="FP.Close"(error in=w205) -> (error out=w204:errorcluster)  [unwired: 2 in, 2 out]
          }
        }
        n66 = Merge Errors(w166, w173) -> (w172:errorcluster)
      }
      frame "Handle Errors" {
        # "Handle Errors. If the Application Manager has started when the error occurred, continue handling events to ensure proper shutdown.  Otherwise, shut down immediately."
        n67 = Unbundle By Name(w214) -> ("Manager Controls.Application Manager"=w212:refnum<k7>)
        n68 = call "Display Error.vi"("error in (no error)"=w215, "Application Manager"=w212) -> ("error out"=w213:errorcluster)  [unwired: 9 out]
        n69 = property class="IApplicationMgr"(reference=w212, error in=w213) -> (error out=w208:errorcluster, "IsStarted"=w211:bool)  [unwired: 1 out]
        n70 = call <vilib>:"Clear Errors.vi"("error in (no error)"=w208) -> ("error out"=w207:errorcluster)  [unwired: 5 in, 1 out]
        n71 = Select(t=State_Selector."Stop" ("Enum"), s=w211, f=State_Selector."Shutdown" ("Enum")) -> (s? t:f=w209:T1)
      }
    }
    "Enum" <- w66
    n72 = call "Check for Errors.vi"("Error In"=w63, "State"=w66) -> ("Error Out"=w64:errorcluster, "State Out"=w65:T1)  [unwired: 8 in]
    "Numeric" <- w62
  }
  n73 = invoke on="Simulator Display" class="Simulator Display (strict)" method="Get Scene Window.vi"() -> ("SceneWindow"=w51:refnum<vi>)  [unwired: 4 in, 3 out]
  n74 = Current VI's Path() -> (path=w55:path)
  n75 = Strip Path(path=w55) -> (stripped path=w54:path)  [unwired: 1 out]
  n76 = Build Path(base path=w54, name or relative path="manifest filename") -> (appended path=w53:path)
  n77 = call <vilib>:"Start Simulator Service.vi"("step mode"=w50, "3D picture refnum"=w51, "step size (ms)"=5.0 ("stepsize(ms)"), "manifest file"=w53) -> ("error out"=w47:errorcluster)  [unwired: 7 in]
  n78 = call <vilib>:"NI VeriStand - Open Workspace Manager Reference.vi"("error in (no error)"=w2, "Gateway IP Address (\"\": localhost)"="localhost" ("Gateway IP Address (\"\": localhost)")) -> ("error out"=w32:errorcluster, "WorkspaceManager"=w33:T7)  [unwired: 8 in]
  n79 = call <instrlib>:"Initialize (Simulator).vi"("error in (no error)"=w47, "Device ID"=T4 {"Robot ID"="N Gear_R0", "Device Label"="Motor_Tire"}) -> ("error out"=w41:errorcluster, "DC Motor Controller out"=w42:refnum<class "DC Motor Controller.lvclass">)  [unwired: 8 in]
  n80 = call <instrlib>:"Initialize (Simulator).vi"("error in (no error)"=w47, "Device ID"=T4 {"Robot ID"="N Gear_R0", "Device Label"="Motor_Arm"}) -> ("error out"=w39:errorcluster, "DC Motor Controller out"=w40:refnum<class "DC Motor Controller.lvclass">)  [unwired: 8 in]
  n81 = while {
    shift-right: [w229] -> w5
    shift-left: w32 -> [w231]
    shift-right: [w226] -> w38
    shift-left: w42 -> [w228]
    shift-right: [w225] -> w37
    shift-left: w41 -> [w221]
    shift-right: [w224] -> w36
    shift-left: w40 -> [w227]
    shift-right: [w223] -> w35
    shift-left: w39 -> [w222]
    shift-right: [w220] -> w34
    shift-left: w33 -> [w219]
    i -> [w216]
    stop <- w218 stop-if-true
    # "Get data from three different channels specified in the System Definition file. Then graph the data."
    n82 = local read "DemoStart"() -> (w217:bool)
    n83 = case shown="True" w217 {
      tunnel: w231 -> [w232 w292]
      tunnel: [w232 w240] -> w229
      tunnel: w228 -> [w237 w291]
      tunnel: w227 -> [w235 w290]
      tunnel: [w237 w289] -> w226
      tunnel: [w236 w288] -> w225
      tunnel: [w235 w287] -> w224
      tunnel: [w234 w286] -> w223
      tunnel: w222 -> [w234 w285]
      tunnel: w221 -> [w236 w284]
      tunnel: [w233 w283] -> w220
      tunnel: w219 -> [w233 w282]
      tunnel: [_ w250] -> w218
      frame False {
      }
      frame True {
        n84 = call-poly <vilib>:"NI VeriStand - Get Channel Value.vi"("error in (no error)"=w292, "Channels"=string[] ["Aliases/Proto LGCU N Resolver", "Aliases/Test LGCU N Resolver", "Targets/Controller/User Channels/UI Gear RealSim Control", "Targets/Controller/Simulation Models/Models/Validate Gear Position/Outports/Valid", "Targets/Controller/Simulation Models/Models/Validate Gear Position/Parameters/Error Limit [Degrees]", "Targets/Controller/User Channels/UI N Gear Control", "Targets/Controller/Simulation Models/Models/Calibrate ECU Torque DutyCycle/Outports/Calibrated ECU Torque DutyCycle", "Targets/Controller/Simulation Models/Models/Calibrate ECU Torque DutyCycle/Parameters/CaliTorque_Bypass Calibration", "Targets/Controller/Simulation Models/Models/Calibrate Gear Position/Parameters/CaliPosition_Bypass Calibration", "Targets/Controller/User Channels/Power"] ("Channel"), "WorkspaceManager in"=w282) -> ("error out"=w240:errorcluster, "Values"=w281:dbl[], "WorkspaceManager out"=w283:T7)  [unwired: 6 in]
        n85 = local read "DemoStop"() -> (w238:bool)
        n86 = Index Array(array=w281) -> (element #1=w254:dbl, element #2=w261:dbl, element #3=w268:dbl, element #4=w270:dbl, element #5=w273:dbl, element #6=w267:dbl, element #7=w258:dbl, element #8=w264:dbl, element #9=w265:dbl, element #10=w251:dbl)  [unwired: 10 in]
        "WFC - torque" <- w258
        "Sim Gear N Position:" <- w261
        "Real Gear N Position:" <- w254
        "LGCU Torque DutyCycle:" <- w258
        "Sim Gear Position [deg]" <- w261
        n87 = Array Subset(array=w281, length=3) -> (w276:dbl[])  [unwired: 1 in]
        n88 = Not Equal To 0?(x=w268) -> (x != 0?=→"Real Gear Enabled":bool)
        n89 = Subtract(x=w261, y=w254) -> (x-y=w266:dbl)
        "Position Error:" <- w266
        n90 = Not Equal To 0?(x=w264) -> (x != 0?=→"Bypass Torque Calibration":bool)
        n91 = Not Equal To 0?(x=w265) -> (x != 0?=→"Bypass Position Calibration":bool)
        n92 = Negate(x=w273) -> (-x=w272:dbl)
        n93 = Subtract(x=1.0, y=w270) -> (x-y=w271:dbl)
        n94 = To Double Precision Float(number=w267) -> (double precision float=w252:dbl)
        "Command" <- w252
        n95 = Build Array (concatenate)(w276) -> (w279:dbl[])
        n96 = Build Array(w266, w273, w272, w271, w270) -> (w278:dbl[])
        n97 = Build Array(w279) -> (→"WFC":dbl[][])
        n98 = Build Array(w278) -> (→"WFC - error":dbl[][])
        n99 = Unbundle By Name(w285) -> ("status"=w241:bool)
        n100 = Unbundle By Name(w284) -> ("status"=w260:bool)
        n101 = Or(x=w240, y=w238) -> (x .or. y?=w239:bool)
        n102 = call "DegreetoSpeed.vi"("Command"=w252, "Torque"=w258) -> ("Numeric"=w256:dbl)  [unwired: 9 in]
        n103 = Compound Arithmetic op=OR(w260, w241) -> (w259:bool)
        n104 = Multiply(x=w256, y=-1.0) -> (x*y=w255:dbl)
        n105 = call-dynamic "Set Velocity Setpoint.vi"("error in (no error)"=w285, "CCW Velocity (0 rad/s)"=w256, "DC Motor Controller in"=w290) -> ("error out"=w286:errorcluster, "DC Motor Controller out"=w287:refnum<class "DC Motor Controller.lvclass">)  [unwired: 7 in]
        n106 = call-dynamic "Set Velocity Setpoint.vi"("error in (no error)"=w284, "CCW Velocity (0 rad/s)"=w255, "DC Motor Controller in"=w291) -> ("error out"=w288:errorcluster, "DC Motor Controller out"=w289:refnum<class "DC Motor Controller.lvclass">)  [unwired: 7 in]
        n107 = Equal To 0?(x=w251) -> (x = 0?=w247:bool)
        n108 = feedback-in #1(w247) -> ()
        n109 = feedback #1(FALSE) -> (w248:bool)
        n110 = Exclusive Or(1:w247, 2:w248) -> (0:w246:bool)
        n111 = feedback #2(0) -> (w244:i32)
        n112 = case shown="False" w246 {
          tunnel: [w295 w297] -> w243
          tunnel: w244 -> [w295 w296]
          frame False {
          }
          frame True {
            n113 = Increment(x=w296) -> (x+1=w297:i32)
          }
        }
        n114 = feedback-in #2(w243) -> ()
        n115 = case shown="3" w243 {
          tunnel: [FALSE TRUE] -> w242
          frame Default {
          }
          frame 3 {
          }
        }
        "读数停止" <- w242
        n116 = Compound Arithmetic op=OR(w242, w259, w239) -> (w250:bool)
      }
    }
    n117 = Wait (ms)(milliseconds to wait=u32 100) -> ()  [unwired: 1 out]
    "Numeric 2" <- w216
  }
  n118 = call <vilib>:"IMAQdx Open Camera.vi"("Session In"=refnum<k21> "cam1" ("Camera Name")) -> ("error out"=w26:errorcluster, "Session Out"=w21:T8)  [unwired: 2 in, 7 out]
  n119 = property class="IMAQdx"(reference=w21, error in=w26, "VideoMode"=w28) -> (reference out=w25:T8, error out=w27:errorcluster)
  n120 = call "IMAQ Create"("Image Name"="Grab") -> ("New Image"=w16:T2)  [unwired: 3 in, 2 out]
  n121 = call <vilib>:"IMAQdx Configure Grab.vi"("error in"=w27, "Session In"=w25) -> ("error out"=w18:errorcluster, "Session Out"=w17:T8)  [unwired: 8 out]
  n122 = while {
    tunnel: [w304] -> w19
    tunnel: w18 -> [w306]
    tunnel: w17 -> [w307]
    tunnel: [w302] -> w20
    tunnel: w16 -> [w305]
    stop <- w301 stop-if-true
    n123 = call <vilib>:"IMAQdx Grab2.vi"("error in"=w306, "Image In"=w305, "Session In"=w307) -> ("error out"=w302:errorcluster, "Buffer Number Out"=w303:u32, "Image Out"=→"Real Gear Position":T2, "Session Out"=w304:T8)  [unwired: 5 in]
    n124 = local read "读数停止"() -> (w298:bool)
    n125 = Get Date/Time In Seconds() -> (seconds since 1Jan1904=→"Time Stamp Control":timestamp)
    n126 = call <vilib>:"Calculate Frames per Second.vi"("Buffer Number"=w303) -> ()  [unwired: 8 in, 3 out]
    n127 = Compound Arithmetic op=OR(w302, w298) -> (w301:bool)
  }
  n128 = call <vilib>:"IMAQdx Close Camera.vi"("error in"=w20, "Session In"=w19) -> ("error out"=w23:errorcluster)  [unwired: 9 out]
  n129 = call "Imaq Dispose"("error in (no error)"=w23) -> ("error out"=w7:errorcluster)  [unwired: 5 in]
  n130 = call-dynamic "Close.vi"("error in (no error)"=w35, "DC Motor Controller in"=w36) -> ("error out"=w46:errorcluster)  [unwired: 9 in]
  n131 = call-dynamic "Close.vi"("error in (no error)"=w37, "DC Motor Controller in"=w38) -> ("error out"=w45:errorcluster)  [unwired: 9 in]
  n132 = Merge Errors(w5, w3) -> (w4:errorcluster)
  n133 = call <vilib>:"NI VeriStand - Close Workspace Manager Reference.vi"("error in (no error)"=w4, "WorkspaceManager"=w34) -> ("error out"=w31:errorcluster)  [unwired: 9 in]
  n134 = flat-sequence {
    tunnel: w31 -> [w309]
    tunnel: [w309] -> w6
    tunnel: [w310] -> w30
    tunnel: w6 -> [w310]
    frame #0 {
      n135 = One Button Dialog(message="Demo Finished!") -> ()  [unwired: 1 in, 1 out]
    }
    frame #1 {
      n136 = for {
        tunnel: u32[] [1, 2] ("Active Plot") -> [w313] mode=indexing
        n137 = property on="WFC - error" class="WFChart (strict)"("Active Plot"=w313, "Plot.Line Style"=u8 2) -> ()  [unwired: 2 in, 2 out]
      }
    }
  }
  n138 = Merge Errors(w7, w45, w46, w30) -> (w1:errorcluster)
  n139 = control-ref of="This VI"() -> (w9:refnum<vi>)
  n140 = call <vilib>:"Stop Simulator Service.vi"("error in (no error)"=w1) -> ("error out"=w10:errorcluster)  [unwired: 10 in]
  n141 = invoke class="VI" method="Default Vals.Reinit All"(reference=w9, error in=w10) -> (error out=w8:errorcluster)  [unwired: 1 in, 2 out]
  "error out" <- w8
  n142 = call <vilib>:"Simple Error Handler.vi"("error in (no error)"=w8) -> ()  [unwired: 4 in, 5 out]
